vi "Precision_Recall_Curve.vi"(8 "error in (no error)":errorcluster caption="entrée d'erreur (pas d'erreur)", 9 "probas_pred":string[][](array[string]), 10 "y_true":string[][](array[string]), 11 "precision_recall_curve":T2={"pos_label"={"dtype_pos_label"="None", "pos_label"="None"}, "sample_weight"=[], "Returns"="precision"}) -> (0 "error out":errorcluster caption="sortie d'erreur", 3 "Data":T1)   [LabVIEW 2020]
doc: "Compute precision-recall pairs for different probability thresholds\n\nNote: this implementation is restricted to the binary classification task.\n\nThe precision is the ratio tp / (tp + fp) where tp is the number of true positives and fp the number of false positives. The precision is intuitively the ability of the classifier not to label as positive a sample that is negative.\n\nThe recall is the ratio tp / (tp + fn) where tp is the number of true positives and fn the number of false negatives. The recall is intuitively the ability of the classifier to find all the positive samples.\n\nThe last precision and recall values are 1. and 0. respectively and do not have a corresponding threshold. This ensures that the graph starts on the y axis.\n\n\n\nParameters : \n\n- y_true : array, shape = [n_samples]\nTrue binary labels. If labels are not either {-1, 1} or {0, 1}, then pos_label should be explicitly given.\n\n- probas_pred : array, shape = [n_samples]\nEstimated probabilities or decision function.\n\n- pos_label : int or str, default=None\nThe label of the positive class. When pos_label=None, if y_true is in {-1, 1} or {0, 1}, pos_label is set to 1, otherwise an error will be raised.\n\n- sample_weight : array-like of shape (n_samples,), default=None\nSample weights.\n\nReturns : \n\n- precision : array, shape = [n_thresholds + 1]\nPrecision values such that element i is the precision of predictions with score >= thresholds[i] and the last element is 1.\n\n- recall : array, shape = [n_thresholds + 1]\nDecreasing recall values such that element i is the recall of predictions with score >= thresholds[i] and the last element is 0.\n\n- thresholds : array, shape = [n_thresholds <= len(np.unique(probas_pred))]\nIncreasing thresholds on the decision function used to compute precision and recall."
uses:
  Precision_Recall_Curve.lvclass
panel:
  out "Precision_Recall_Curve.lvclass":refnum<class "Precision_Recall_Curve.lvclass">
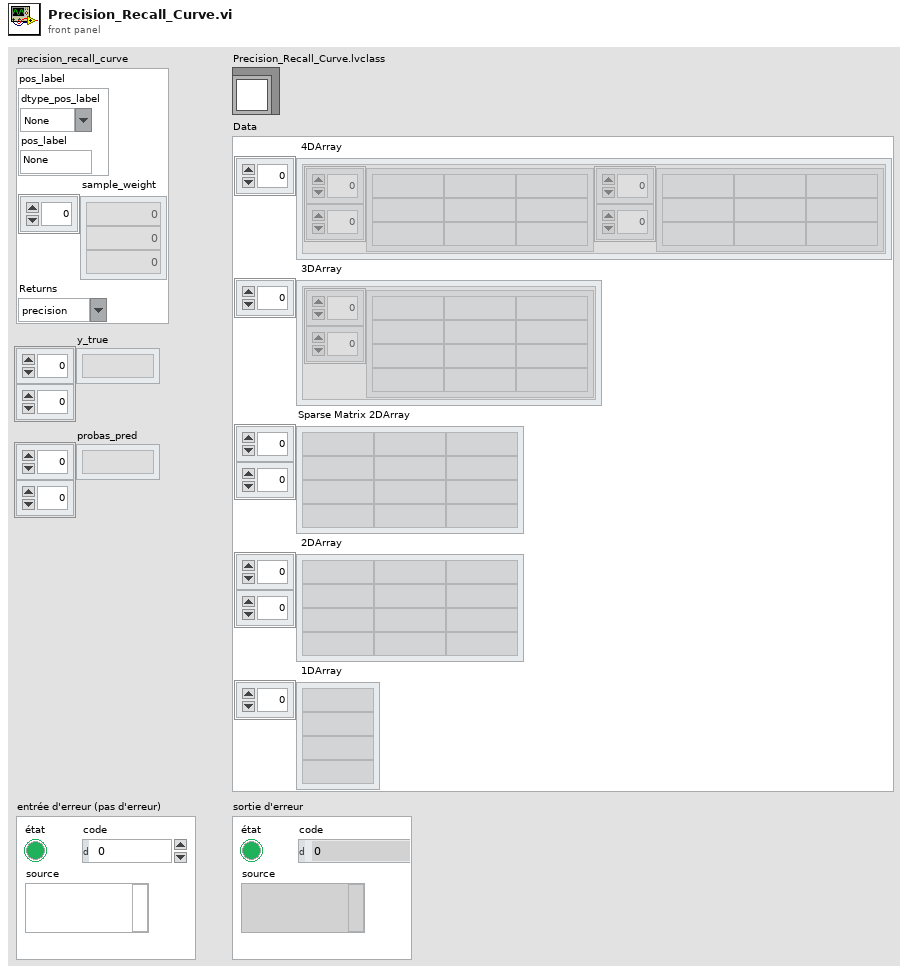
[diagram p1: front panel]
types:
  T1 = cluster{" 4DArray":cluster{"1":string[][], "2":string[][]}[], " 3DArray":cluster{"Tableau":string[][]}[], "Sparse Matrix 2DArray":string[][], " 2DArray":string[][], " 1DArray":string[]}
  T2 = cluster{"pos_label":cluster{"dtype_pos_label":string, "pos_label":string}, "sample_weight":dbl[], "Returns":string}
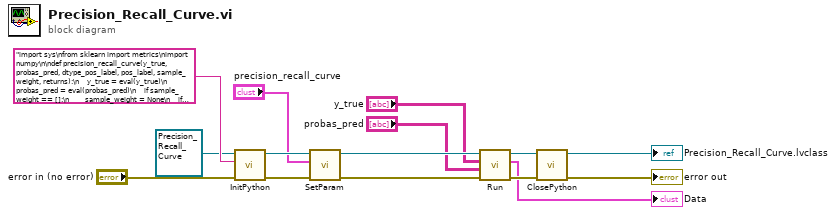
[diagram p0: block diagram]
diagram:
  n1 = call-dynamic "InitPython.vi"("error in (no error)"="error in (no error)", "Python Instruction"="import sys\nfrom sklearn import metrics\nimport numpy\n\ndef precision_recall_curve(y_true, probas_pred, dtype_pos_label, pos_label, sample_weight, returns):\n    y_true = eval(y_true)\n    probas_pred = eval(probas_pred)\n    if sample_weight == []:\n        sample_weight = None\n    if dtype_pos_label == 'int':\n        pos_label = eval(pos_label)\n    elif dtype_pos_label == 'None':\n        pos_label = None\n    try:\n        precision, recall, thresholds = metrics.precision_recall_curve(y_true, probas_pred, pos_label, sample_weight)\n        if returns == 'precision':\n            precision_recall_curve = precision.tolist()\n            return str(precision_recall_curve)\n        elif returns == 'recall':\n            precision_recall_curve = recall.tolist()\n            return str(precision_recall_curve)\n        else:\n            precision_recall_curve = thresholds.tolist()\n            return str(precision_recall_curve)\n    except:\n        erreur = sys.exc_info()\n        typerr = u\"%s\" % (erreur[0])\n        typerr = typerr[typerr.find(\"'\")+1:typerr.rfind(\"'\")]\n        msgerr = u\"%s\" % (erreur[1])\n        message = str('/!\\\\ {0} : {1}'. format(typerr,msgerr))\n        return message", "Scikit-learn en entrée"=refnum<class "Precision_Recall_Curve.lvclass"> refnum ("Precision_Recall_Curve.lvclass")) -> ("error out"=w11:errorcluster, "Scikit-learn en sortie"=w12:refnum<class "Precision_Recall_Curve.lvclass">)  [unwired: 7 in]
  n2 = call-dynamic "SetParam.vi"("error in (no error)"=w11, "precision_recall_curve"="precision_recall_curve", "Precision_Recall_Curve.lvclass"=w12) -> ("error out"=w8:errorcluster, "Precision_Recall_Curve.lvclass"=w9:refnum<class "Precision_Recall_Curve.lvclass">)  [unwired: 7 in]
  n3 = call-dynamic "Run.vi"("error in (no error)"=w8, "probas_pred"="probas_pred", "y_true"="y_true", "Precision_Recall_Curve.lvclass"=w9) -> ("error out"=w6:errorcluster, "Data"=→"Data":T1, "Precision_Recall_Curve.lvclass"=w7:refnum<class "Precision_Recall_Curve.lvclass">)  [unwired: 5 in]
  n4 = call-dynamic "ClosePython.vi"("error in (no error)"=w6, "Scikit-learn en entrée"=w7) -> ("error out"=→"error out":errorcluster, "Scikit-learn en sortie"=→"Precision_Recall_Curve.lvclass":refnum<class "Precision_Recall_Curve.lvclass">)  [unwired: 8 in]
